vi "delay.vi"(8 "valor delay":u32=300, 9 "element":T1(ring), 10 "arreglo opciones":bool[](array[boolean])=[FALSE, FALSE, FALSE, FALSE]) -> ()   [LabVIEW 2016]
doc: "Este subVI es el que indica el tamaño del delay de acuerdo al tamaño de este en milisegundos."
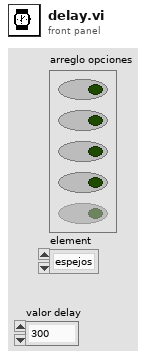
[diagram p1: front panel]
types:
  T1 = enum16{"espejos", "polarizador", "voltaje", "potenciometro y lockin", "CCD"}
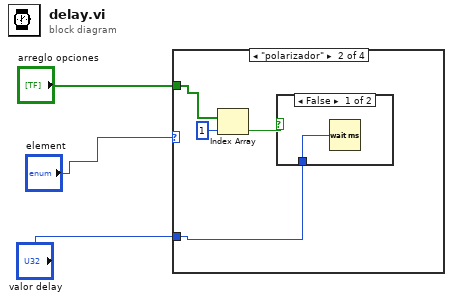
[diagram p0: block diagram]
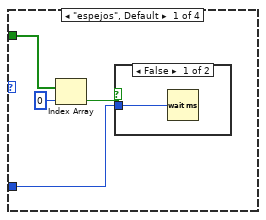
[diagram p2: hidden frame]
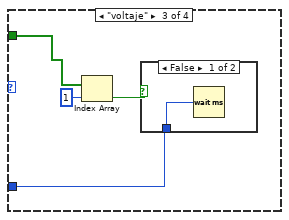
[diagram p5: hidden frame]
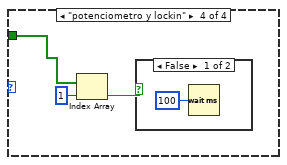
[diagram p7: hidden frame]
diagram:
  n1 = case shown="\"polarizador\"" "element" {
    tunnel: "arreglo opciones" -> [w6 w12 w15 w19]
    tunnel: "valor delay" -> [w4 w9 w14 _]
    frame "espejos", Default {
      n2 = Index Array(array=w6, index=0) -> (element=w7:bool)
      n3 = case shown="False" w7 {
        tunnel: w4 -> [w8 _]
        frame False {
          n4 = Wait (ms)(milliseconds to wait=w8) -> ()  [unwired: 1 out]
        }
        frame True {
        }
      }
    }
    frame "polarizador" {
      n5 = Index Array(array=w12, index=1) -> (element=w10:bool)
      n6 = case shown="False" w10 {
        tunnel: w9 -> [w13 _]
        frame False {
          n7 = Wait (ms)(milliseconds to wait=w13) -> ()  [unwired: 1 out]
        }
        frame True {
        }
      }
    }
    frame "voltaje" {
      n8 = Index Array(array=w15, index=1) -> (element=w16:bool)
      n9 = case shown="False" w16 {
        tunnel: w14 -> [w18 _]
        frame False {
          n10 = Wait (ms)(milliseconds to wait=w18) -> ()  [unwired: 1 out]
        }
        frame True {
        }
      }
    }
    frame "potenciometro y lockin" {
      n11 = Index Array(array=w19, index=1) -> (element=w20:bool)
      n12 = case shown="False" w20 {
        frame False {
          n13 = Wait (ms)(milliseconds to wait=u32 100) -> ()  [unwired: 1 out]
        }
        frame True {
        }
      }
    }
  }
